vi "Read and Write Controls to Automatic Config File.vi"(4 "path":path, 6 "Use Path":bool, 7 "Action":T1, 8 "error in":errorcluster, 10 "Control References":refnum<vi>[](array[refnum])) -> (0 "error out":errorcluster, 3 "ctrl file path":path)   [LabVIEW 2018]
doc: "Writes the values of an array of controls to a configuration file or reads them back.\n<b>Control References</b> is an array of the references of the controls to be saved.\n\nThe configuration file is named after the VI the first control in the array is in and is saved in the LabVIEW Data folder"
uses:
  RWC_Actions.ctl
  <vilib>/Utility/config.llb/NI_LVConfig.lvlib
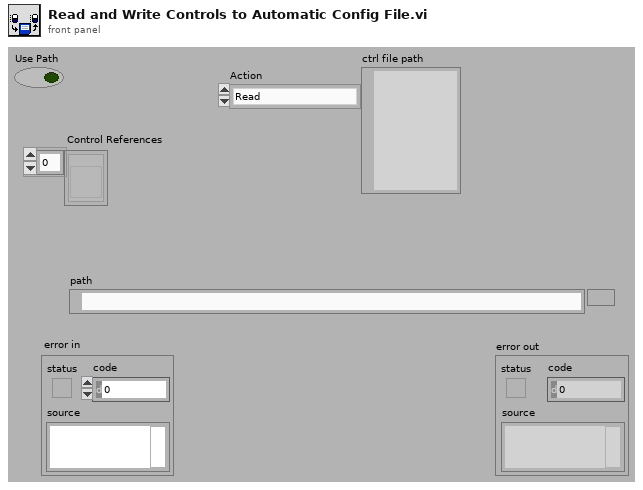
[diagram p1: front panel]
types:
  T1 = typedef "RWC_Actions.ctl" = enum16{"Read", "Write", "Read and Create"}
  T2 = typedef "NI_LVConfig.lvlib/Config Data RefNum.ctl" = refnum<k1>
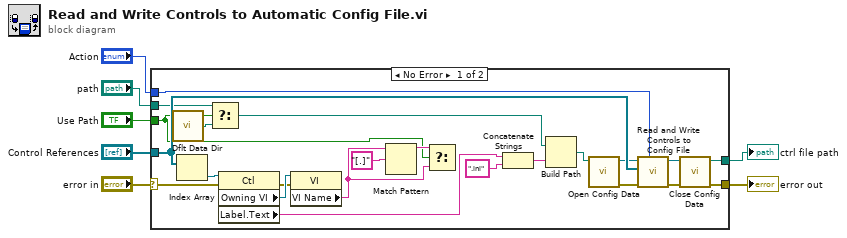
[diagram p0: block diagram]
diagram:
  n1 = case shown="No Error" "error in" {
    selector: "error in" -> [w20 w31]
    tunnel: "Action" -> [w30 _]
    tunnel: "Control References" -> [w29 _]
    tunnel: [w21 w31] -> w4
    tunnel: "Use Path" -> [w10 _]
    tunnel: "path" -> [w15 _]
    tunnel: [w17 _] -> w1
    frame No Error {
      n2 = call <vilib>:"Dflt Data Dir.vi"() -> ("App:Default Data Directory"=w16:path)
      n3 = Index Array(array=w29) -> (element=w9:refnum<vi>)  [unwired: 1 in]
      n4 = Select(t=w15, s=w10, f=w16) -> (s? t:f=w18:path)
      n5 = property class="Ctl"(reference=w9, error in=w20) -> (error out=w26:errorcluster, "Owning VI"=w28:refnum<vi>, "Label.Text"=w8:string)  [unwired: 1 out]
      n6 = property class="VI"(reference=w28, error in=w26) -> ("VI Name"=w11:string)  [unwired: 2 out]
      n7 = Match Pattern(string=w11, regular expression="[.]") -> (before substring=w12:string)  [unwired: 1 in, 3 out]
      n8 = Select(t=w12, s=w10, f=w11) -> ()  [unwired: 1 out]
      n9 = Concatenate Strings(w8, ".ini" ("string")) -> (w27:string)
      n10 = Build Path(base path=w18, name or relative path=w27) -> (appended path=w19:path)
      n11 = call <vilib>:"Open Config Data.vi"("configuration file path"=w19) -> ("error out"=w25:errorcluster, "refnum"=w23:T2)  [unwired: 8 in, 1 out]
      n12 = call "Read and Write Controls to Config File.vi"("Action"=w30, "error in"=w25, "Control References"=w29, "Configuration File Reference In"=w23) -> ("error out"=w22:errorcluster, "Configuration File Reference Out"=w24:T2)  [unwired: 6 in]
      n13 = call <vilib>:"Close Config Data.vi"("error in (no error)"=w22, "refnum"=w24) -> ("error out"=w21:errorcluster, "file path"=w17:path)  [unwired: 8 in]
    }
    frame Error {
    }
  }
  "error out" <- w4
  "ctrl file path" <- w1
